vi "PC_AINoiseMeas.vi"() -> ()   [LabVIEW 2020]
uses:
  TypeDefs/UIStateDefEnum.ctl
  <vilib>/measure/maspectr.llb/Power Spectrum and PSD Export Mode.ctl
  <vilib>/Analysis/baseanly.llb/Mean (DBL).vi
  <vilib>/Analysis/5stat.llb/RMS (DBL).vi
  <vilib>/NI/STM/TCP/Read Meta Data (TCP Ref).vi
  <vilib>/NI/STM/TCP/Get Connection Reference (TCP).vi
  <vilib>/measure/maspectr.llb/FFT Power Spectrum and PSD for 1 Chan.vi
  <vilib>/Analysis/1siggen.llb/Ramp Pattern by Delta.vi
  <vilib>/Utility/file.llb/Write Delimited Spreadsheet (DBL).vi
  <vilib>/NI/STM/TCP/Read Meta Data (TCP Clst).vi
  <vilib>/NI/STM/TCP/Read Message (TCP).vi
  <vilib>/NI/STM/NI STM.lvlib
  <vilib>/Analysis/NI_AALBase.lvlib
  <vilib>/measure/NI_MAPro.lvlib
  <vilib>/Analysis/NI_AALPro.lvlib
  Components_global/Spectra/Spectra.lvlib
panel:
  in  "STM LoopTime Set [ms]":u32=100
  in  "Save Data":bool
  out "Analysis Loop \ntime [s]":dbl format="%#.4g"
  out "Analysis \ntime-span [s]":dbl format="%.2f"
  out "# of elements \nremoved":i32
  in  "Pause Charts":bool
  in  "Clear charts":bool
  out "RT target \nloop \ntime [s]":dbl=0.0002
  out "Data length \n[count]":i32
  out "Mean [V]":dbl format="%#.6f"
  out "RMS / \nStd. Dev. [mV]":dbl format="%#.6f"
  out "Spectra plots":cluster{"f0":dbl, "df":dbl, "magnitude":dbl[]}[](graph)
  out "Histogram Graph":T1(graph)
  out "STM Loop \ntime [s]":dbl format="%#.4g"
  in  "System Stop Button":bool
  out "Data":dbl[][](graph)
  # "Hidden Controls and Indicators"
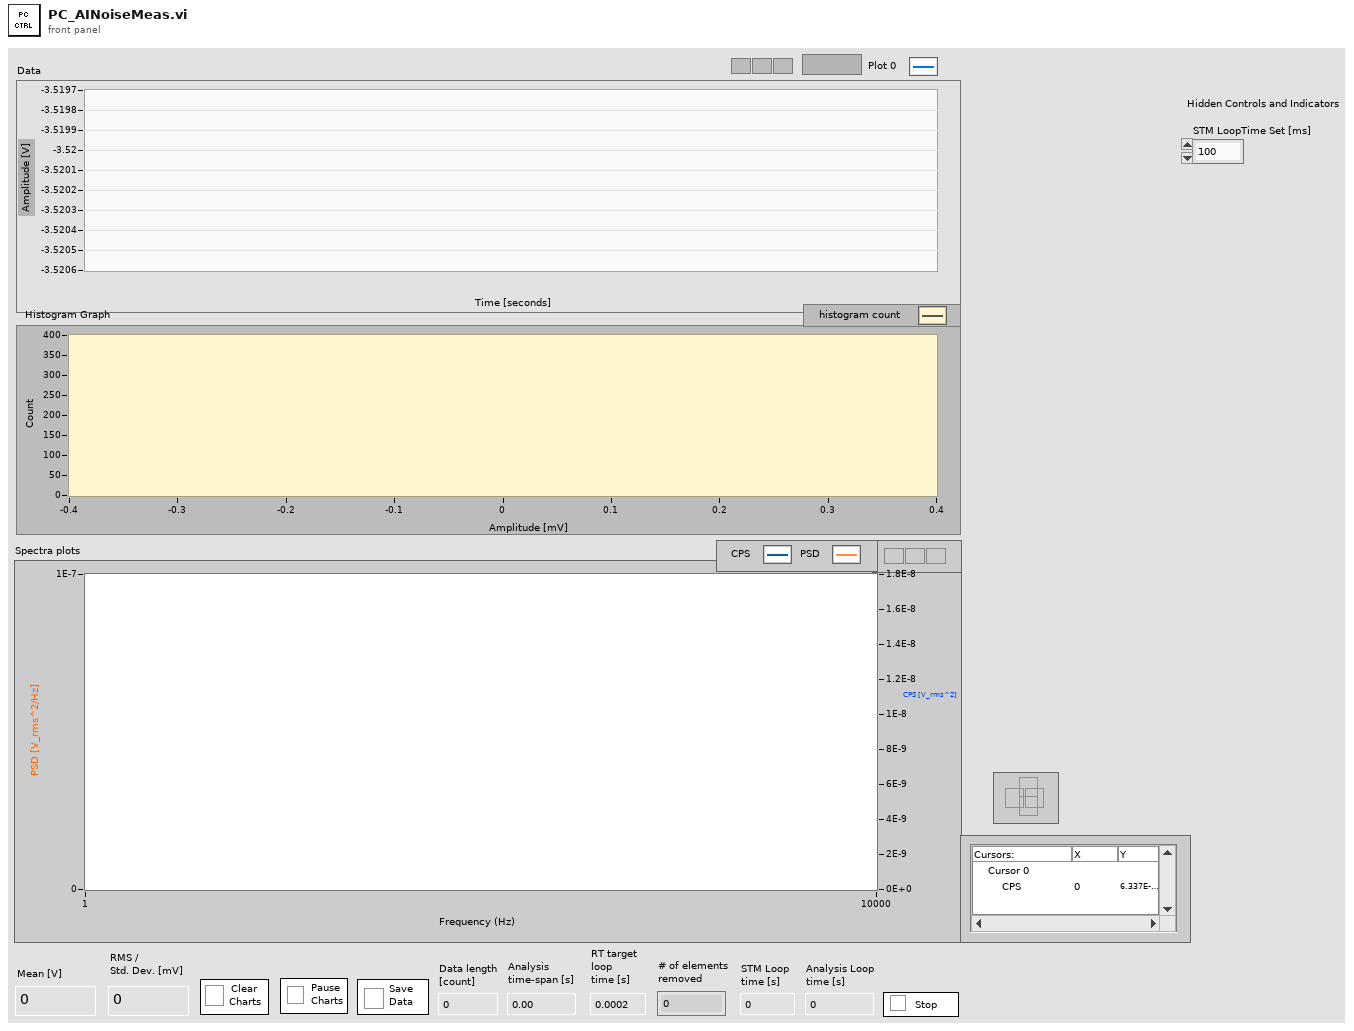
[diagram p1: front panel]
types:
  T1 = cluster{"X Values":dbl[], "Histogram: h(x)":i32[]}
  T2 = typedef "UIStateDefEnum.ctl" = enum16{"Wait", "Initialize", "Clear", "SaveData", "Stop"}
  T3 = typedef "NI STM.lvlib/TCP Connection Info.ctl" = cluster{"connection ID":refnum<k5>, "meta data":T4[]}
  T4 = typedef "NI STM.lvlib/MetaDataElement.ctl" = string
  T5 = typedef "NI_MAPro.lvlib/Power Spectrum and PSD Export Mode.ctl" = u16
  T6 = typedef "imagedata.ctl" = cluster{"image type":i32, "image depth":i32, "image":u8[], "mask":u8[], "colors":u32[], "Rectangle":cluster{"left":i16, "top":i16, "right":i16, "bottom":i16}}
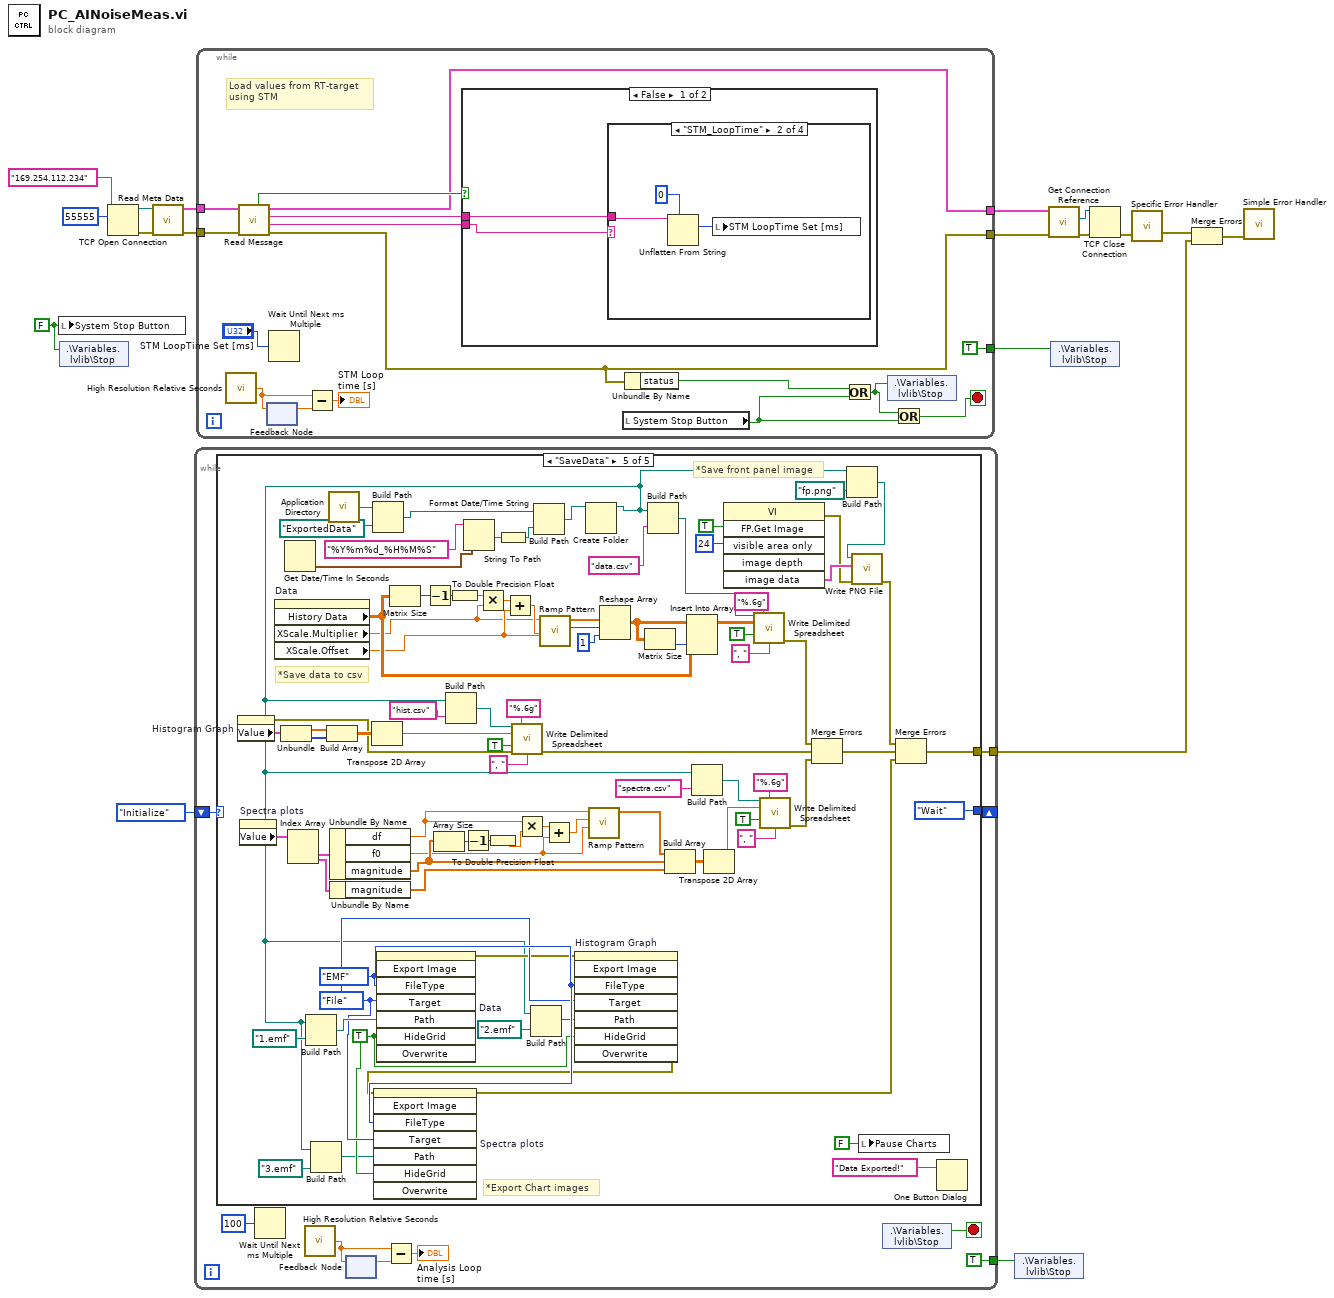
[diagram p0: block diagram]
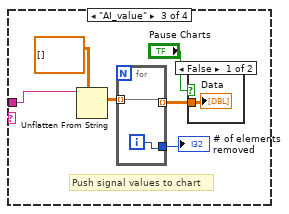
[diagram p3: hidden frame]
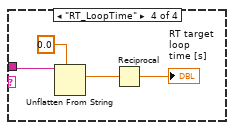
[diagram p5: hidden frame]
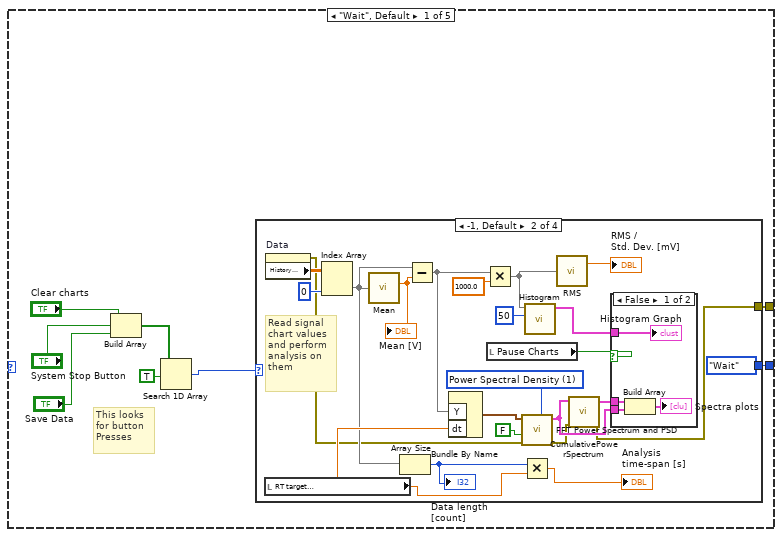
[diagram p7: hidden frame]
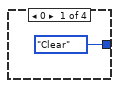
[diagram p8: hidden frame]
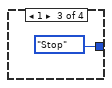
[diagram p10: hidden frame]
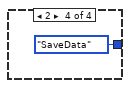
[diagram p11: hidden frame]
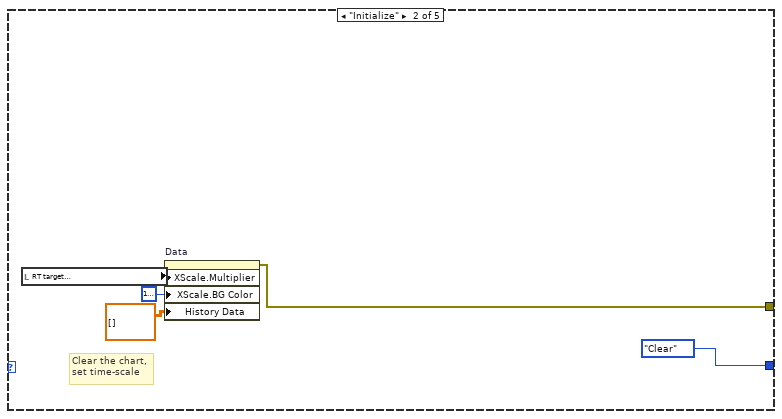
[diagram p12: hidden frame]
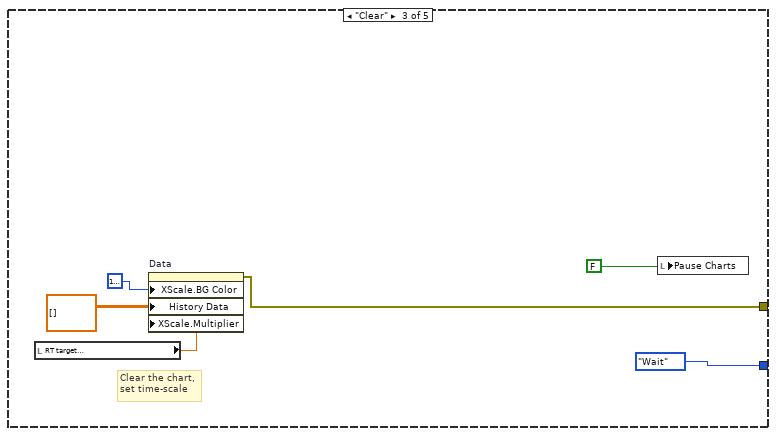
[diagram p13: hidden frame]
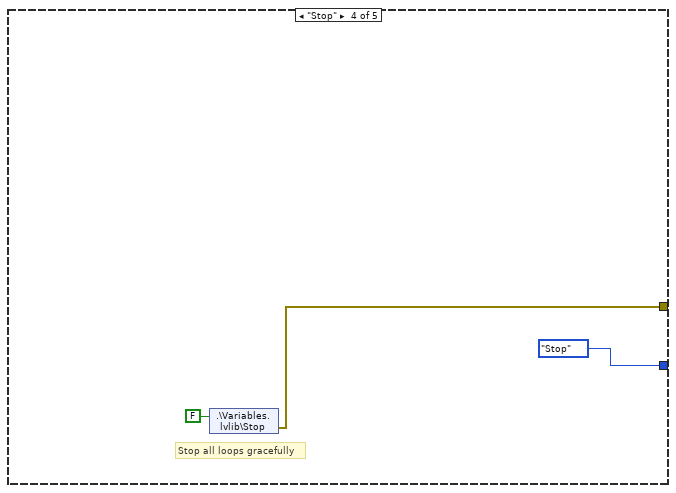
[diagram p14: hidden frame]
diagram:
  w7 = FALSE ("System Stop Button")
  n1 = local write "System Stop Button"(w7) -> ()
  n2 = shared-variable ".\\Variables.lvlib\\Stop"(w7) -> ()  [unwired: 1 in, 1 out]
  n3 = TCP Open Connection(address="169.254.112.234", remote port or service name=u16 55555) -> (connection ID=w16:refnum<k5>, error out=w15:errorcluster)  [unwired: 3 in]
  n4 = call-poly <vilib>:"Read Meta Data.vi"("error in"=w15, "connection ID"=w16) -> ("error out"=w13:errorcluster, "connection info out"=w14:T3)  [unwired: 7 in, 1 out]
  n5 = while {
    shift-right: [w25] -> _
    shift-left: UIStateDefEnum."Initialize" ("UIStateDefEnum") -> [w26]
    tunnel: [w20] -> w2
    tunnel: [TRUE ("Stop")] -> w1
    stop <- w24 stop-if-true
    n6 = case shown="\"SaveData\"" w26 {
      tunnel: [w30 UIStateDefEnum."Clear" ("UIStateDefEnum") UIStateDefEnum."Wait" ("UIStateDefEnum") UIStateDefEnum."Stop" ("UIStateDefEnum") UIStateDefEnum."Wait" ("UIStateDefEnum")] -> w25
      tunnel: [w28 w66 w71 w77 w120] -> w20
      frame "Wait", Default {
        # "This looks \nfor button \nPresses"
        n7 = Build Array "Build Array"("Clear charts", "System Stop Button", "Save Data") -> (w35:bool[])
        n8 = Search 1D Array(1D array=w35, element=TRUE) -> (index of element=w31:i32)  [unwired: 1 in]
        n9 = case shown="-1, Default" w31 {
          tunnel: [UIStateDefEnum."Clear" ("UIStateDefEnum") UIStateDefEnum."Wait" ("UIStateDefEnum") UIStateDefEnum."Stop" ("UIStateDefEnum") UIStateDefEnum."SaveData" ("UIStateDefEnum")] -> w30
          tunnel: [_ w37 _ _] -> w28
          frame 0 {
          }
          frame -1, Default {
            w55 = T5 1 items=["Power Spectrum", "Power Spectral Density"] ("export mode")
            # "Read signal\nchart values\nand perform\nanalysis on \nthem"
            n10 = local read "RT target \nloop \ntime [s]"() -> (w48:dbl)
            n11 = property on="Data" class="WFChart (strict)"() -> (error out=w38:errorcluster, "History Data"=w53:dbl[][])  [unwired: 2 in, 1 out]
            n12 = Index Array(array=w53, index (col)=0 ("disabled index (col)")) -> (element=w43:dbl[])  [unwired: 1 in]
            n13 = call-poly <vilib>:"Mean.vi"("X"=w43) -> ("mean"=w54:dbl)  [unwired: 1 out]
            "Mean [V]" <- w54
            n14 = Array Size(array=w43) -> (size(s)=w49:i32)
            "Data length \n[count]" <- w49
            n15 = Subtract(x=w43, y=w54) -> (x-y=w42:dbl[])
            n16 = Bundle By Name("Y"=w42, "dt"=w48) -> (w57:waveform(dbl))  [unwired: 1 in]
            n17 = Multiply(x=w42, y=1000.0) -> (x*y=w44:dbl[])
            n18 = local read "Pause Charts"() -> (w47:bool)
            n19 = call-poly <vilib>:"FFT Power Spectrum and PSD.vi"("export mode"=w55, "error in (no error)"=w38, "dB On (F)"=FALSE, "time signal"=w57) -> ("error out"=w39:errorcluster, "Power Spectrum / PSD"=w40:cluster{"f0":dbl, "df":dbl, "magnitude":dbl[]})  [unwired: 4 in, 2 out]
            n20 = Multiply(x=w49, y=w48) -> (x*y=→"Analysis \ntime-span [s]":dbl)
            n21 = call <vilib>:"Histogram.vi"("intervals"=50, "X"=w44) -> ("Histogram Graph"=w58:T1)  [unwired: 6 in, 3 out]
            n22 = call-poly <vilib>:"RMS.vi"("X"=w44) -> ("rms value"=→"RMS / \nStd. Dev. [mV]":dbl)  [unwired: 1 out]
            n23 = call "CumulativePowerSpectrum.vi"("error in (no error)"=w39, "PSD"=w40) -> ("error out"=w37:errorcluster, "CPS"=w41:cluster{"f0":dbl, "df":dbl, "magnitude":dbl[]})  [unwired: 8 in]
            n24 = case shown="False" w47 {
              tunnel: w58 -> [w63 _]
              tunnel: w41 -> [w62 _]
              tunnel: w40 -> [w60 _]
              frame False {
                n25 = Build Array(w62, w60) -> (→"Spectra plots":cluster{"f0":dbl, "df":dbl, "magnitude":dbl[]}[])
                "Histogram Graph" <- w63
              }
              frame True {
              }
            }
          }
          frame 1 {
          }
          frame 2 {
          }
        }
      }
      frame "Initialize" {
        # "Clear the chart,\nset time-scale"
        n26 = local read "RT target \nloop \ntime [s]"() -> (w69:dbl)
        n27 = property on="Data" class="WFChart (strict)"("XScale.Multiplier"=w69, "XScale.BG Color"=u32 16777216 ("X Scale.Marker Colors:BG Color"), "History Data"=dbl[][] []) -> (error out=w66:errorcluster)  [unwired: 2 in, 1 out]
      }
      frame "Clear" {
        # "Clear the chart,\nset time-scale"
        n28 = local read "RT target \nloop \ntime [s]"() -> (w72:dbl)
        n29 = property on="Data" class="WFChart (strict)"("XScale.BG Color"=u32 16777216 ("X Scale.Marker Colors:BG Color"), "History Data"=dbl[][] [], "XScale.Multiplier"=w72) -> (error out=w71:errorcluster)  [unwired: 2 in, 1 out]
        n30 = local write "Pause Charts"(FALSE ("Pause Charts")) -> ()
      }
      frame "Stop" {
        # "Stop all loops gracefully"
        n31 = shared-variable ".\\Variables.lvlib\\Stop"(FALSE ("Stop")) -> (error out=w77:errorcluster)  [unwired: 1 in]
      }
      frame "SaveData" {
        w133 = TRUE ("Hide Grid")
        w136 = enum32{"File", "Clipboard"}."File" ("Target")
        w137 = enum32{"BMP", "EPS", "EMF", "PICT"}."EMF" ("File Type")
        # "*Export Chart images"
        # "*Save front panel image"
        # "*Save data to csv"
        n32 = property on="Histogram Graph" class="XYGraph (strict)"() -> (error out=w91:errorcluster, "Value"=w117:T1)  [unwired: 2 in, 1 out]
        n33 = property on="Spectra plots" class="WFGraph (strict)"() -> ("Value"=w113:cluster{"f0":dbl, "df":dbl, "magnitude":dbl[]}[])  [unwired: 2 in, 2 out]
        n34 = property on="Data" class="WFChart (strict)"() -> ("History Data"=w161:dbl[][], "XScale.Multiplier"=w151:dbl, "XScale.Offset"=w156:dbl)  [unwired: 2 in, 2 out]
        n35 = Unbundle(w117) -> ("X Values"=w116:dbl[], "Histogram: h(x)"=w115:i32[])
        n36 = Get Date/Time In Seconds() -> (seconds since 1Jan1904=w148:timestamp)
        n37 = Index Array(array=w113) -> (element #1=w112:cluster{"f0":dbl, "df":dbl, "magnitude":dbl[]}, element #2=w111:cluster{"f0":dbl, "df":dbl, "magnitude":dbl[]})  [unwired: 2 in]
        n38 = Build Array(w116, w115) -> (w114:dbl[][])
        n39 = call <vilib>:"Application Directory.vi"() -> ("Application Directory"=w150:path)
        n40 = Unbundle By Name(w112) -> ("df"=w105:dbl, "f0"=w103:dbl, "magnitude"=w108:dbl[])
        n41 = Unbundle By Name(w111) -> ("magnitude"=w110:dbl[])
        n42 = Transpose 2D Array(2D array=w114) -> (transposed array=w92:dbl[][])
        n43 = Build Path(base path=w150, name or relative path=path "ExportedData") -> (appended path=w145:path)
        n44 = Matrix Size(0:w161) -> (1:w160:i32)  [unwired: 1 out]
        n45 = Decrement(x=w160) -> (x-1=w159:i32)
        n46 = Array Size(array=w108) -> (size(s)=w100:i32)
        n47 = To Double Precision Float(number=w159) -> (double precision float=w158:dbl)
        n48 = Decrement(x=w100) -> (x-1=w107:i32)
        n49 = Format Date/Time String(time format string (%c)="%Y%m%d_%H%M%S", seconds (now)=w148) -> (date/time string=w143:string)  [unwired: 1 in]
        n50 = Multiply(x=w158, y=w151) -> (x*y=w157:dbl)
        n51 = To Double Precision Float(number=w107) -> (double precision float=w106:dbl)
        n52 = String To Path(string=w143) -> (path=w144:path)
        n53 = Add(x=w157, y=w156) -> (x+y=w155:dbl)
        n54 = Multiply(x=w105, y=w106) -> (x*y=w104:dbl)
        n55 = Build Path(base path=w145, name or relative path=w144) -> (appended path=w138:path)
        n56 = call-poly <vilib>:"Ramp Pattern.vi"("start"=w156, "end"=w155, "delta"=w151) -> ("samples"=w154:i32, "Ramp Pattern"=w153:dbl[])  [unwired: 6 in, 1 out]
        n57 = Add(x=w104, y=w103) -> (x+y=w102:dbl)
        n58 = Create Folder(path (use dialog)=w138) -> (created path=w82:path)  [unwired: 2 in, 2 out]
        n59 = Build Path(base path=w82, name or relative path=path "1.emf") -> (appended path=w141:path)
        n60 = Build Path(base path=w82, name or relative path=path "3.emf") -> (appended path=w132:path)
        n61 = invoke on="Data" class="WFChart (strict)" method="Export Image"("FileType"=w137, "Target"=w136, "Path"=w141, "HideGrid"=w133) -> (error out=w130:errorcluster)  [unwired: 4 in, 7 out]
        n62 = Build Path(base path=w82, name or relative path="hist.csv" ("string")) -> (appended path=w93:path)
        n63 = call-poly <vilib>:"Write Delimited Spreadsheet.vi"("file path (dialog if empty)"=w93, "format (%.3f)"="%.6g", "2D data"=w92, "append to file? (new file:F)"=TRUE, "error in (no error)"=w91, "delimiter (\\t)"=", " ("delimiter (\\t)")) -> ("error out"=w89:errorcluster)  [unwired: 8 in, 1 out]
        n64 = Build Path(base path=w82, name or relative path=path "2.emf") -> (appended path=w135:path)
        n65 = invoke on="Histogram Graph" class="XYGraph (strict)" method="Export Image"(error in=w130, "FileType"=w137, "Target"=w136, "Path"=w135, "HideGrid"=w133) -> (error out=w129:errorcluster)  [unwired: 3 in, 7 out]
        n66 = invoke on="Spectra plots" class="WFGraph (strict)" method="Export Image"(error in=w129, "FileType"=w137, "Target"=w136, "Path"=w132, "HideGrid"=w133) -> (error out=w109:errorcluster)  [unwired: 3 in, 7 out]
        n67 = call-poly <vilib>:"Ramp Pattern.vi"("start"=w103, "end"=w102, "delta"=w105) -> ("Ramp Pattern"=w101:dbl[])  [unwired: 6 in, 2 out]
        n68 = Reshape Array(w153, w154, 1 ("dimension size")) -> (w152:dbl[][])
        n69 = Matrix Size(0:w152) -> (2:w163:i32)  [unwired: 1 out]
        n70 = Build Path(base path=w82, name or relative path="data.csv" ("string")) -> (appended path=w146:path)
        n71 = Build Array(w101, w108, w110) -> (w99:dbl[][])
        n72 = Insert Into Array(array=w152, index (col)=w163, new element=w161) -> (w98:dbl[][])  [unwired: 1 in]
        n73 = Build Path(base path=w82, name or relative path="spectra.csv" ("string")) -> (appended path=w87:path)
        n74 = Transpose 2D Array(2D array=w99) -> (transposed array=w81:dbl[][])
        n75 = invoke class="VI" method="FP.Get Image"("visible area only"=TRUE ("Visible Area Only"), "image depth"=24 ("Image Depth")) -> (error out=w124:errorcluster, "image data"=w126:T6)  [unwired: 4 in, 4 out]
        n76 = call-poly <vilib>:"Write Delimited Spreadsheet.vi"("file path (dialog if empty)"=w146, "format (%.3f)"="%.6g", "2D data"=w98, "append to file? (new file:F)"=TRUE, "delimiter (\\t)"=", " ("delimiter (\\t)")) -> ("error out"=w90:errorcluster)  [unwired: 9 in, 1 out]
        n77 = call-poly <vilib>:"Write Delimited Spreadsheet.vi"("file path (dialog if empty)"=w87, "format (%.3f)"="%.6g", "2D data"=w81, "append to file? (new file:F)"=TRUE, "delimiter (\\t)"=", " ("delimiter (\\t)")) -> ("error out"=w80:errorcluster)  [unwired: 9 in, 1 out]
        n78 = Merge Errors(w90, w89, w80) -> (w88:errorcluster)
        n79 = Build Path(base path=w82, name or relative path=path "fp.png") -> (appended path=w125:path)
        n80 = call <vilib>:"Write PNG File.vi"("error in (no error)"=w124, "image data"=w126, "path to PNG file"=w125) -> ("error out"=w122:errorcluster)  [unwired: 7 in, 1 out]
        n81 = local write "Pause Charts"(FALSE ("Pause Charts")) -> ()
        n82 = Merge Errors(w122, w88, w109) -> (w120:errorcluster)
        n83 = One Button Dialog(message="Data Exported!" ("Status....")) -> ()  [unwired: 1 in, 1 out]
      }
    }
    n84 = Wait Until Next ms Multiple(millisecond multiple=u32 100) -> ()  [unwired: 1 out]
    n85 = call <vilib>:"High Resolution Relative Seconds.vi"() -> ("relative seconds"=w22:dbl)
    n86 = feedback #1() -> (w23:dbl)  [unwired: 1 in]
    n87 = feedback-in #1(w22) -> ()
    n88 = Subtract(x=w22, y=w23) -> (x-y=→"Analysis Loop \ntime [s]":dbl)
    n89 = shared-variable ".\\Variables.lvlib\\Stop"() -> (w24:bool)  [unwired: 1 in, 1 out]
  }
  n90 = while {
    tunnel: w14 -> [w181]
    tunnel: w13 -> [w180]
    tunnel: [w178] -> w9
    tunnel: [w177] -> w8
    tunnel: [TRUE ("Stop")] -> w5
    stop <- w171 stop-if-true
    # "Load values from RT-target\nusing STM"
    n91 = call <vilib>:"High Resolution Relative Seconds.vi"() -> ("relative seconds"=w173:dbl)
    n92 = call-poly <vilib>:"Read Message.vi"("error in"=w180, "connection info in"=w181) -> ("error out"=w177:errorcluster, "name"=w176:T4, "data string"=w175:string, "connection info out"=w178:T3, "timed out?"=w179:bool)  [unwired: 4 in, 1 out]
    n93 = feedback-in #2(w173) -> ()
    n94 = feedback #2() -> (w174:dbl)  [unwired: 1 in]
    n95 = Wait Until Next ms Multiple(millisecond multiple="STM LoopTime Set [ms]") -> ()  [unwired: 1 out]
    n96 = Subtract(x=w173, y=w174) -> (x-y=→"STM Loop \ntime [s]":dbl)
    n97 = case shown="False" w179 {
      tunnel: w176 -> [w183 _]
      tunnel: w175 -> [w182 _]
      frame False {
        n98 = case shown="\"STM_LoopTime\"" w183 {
          tunnel: w182 -> [_ w185 w191 w196]
          frame Default {
          }
          frame "STM_LoopTime" {
            n99 = Unflatten From String(type=u32 0, binary string=w185) -> (value=w184:u32)  [unwired: 3 in, 2 out]
            n100 = local write "STM LoopTime Set [ms]"(w184) -> ()
          }
          frame "AI_value" {
            # "Push signal values to chart"
            n101 = Unflatten From String(type=dbl[][] [], binary string=w191) -> (value=w190:dbl[][])  [unwired: 3 in, 2 out]
            n102 = for {
              tunnel: w190 -> [w195] mode=indexing
              tunnel: [w195] -> w189 mode=indexing
              tunnel: [w194] -> w188
              i -> [w194]
            }
            "# of elements \nremoved" <- w188
            n103 = case shown="False" "Pause Charts" {
              tunnel: w189 -> [w193 _]
              frame False {
                "Data" <- w193
              }
              frame True {
              }
            }
          }
          frame "RT_LoopTime" {
            n104 = Unflatten From String(type=0.0, binary string=w196) -> (value=w198:dbl)  [unwired: 3 in, 2 out]
            n105 = Reciprocal(x=w198) -> (1/x=→"RT target \nloop \ntime [s]":dbl)
          }
        }
      }
      frame True {
      }
    }
    n106 = local read "System Stop Button"() -> (w170:bool)
    n107 = Unbundle By Name(w177) -> ("status"=w169:bool)
    n108 = Or(x=w169, y=w170) -> (x .or. y?=w168:bool)
    n109 = shared-variable ".\\Variables.lvlib\\Stop"(w168) -> ()  [unwired: 1 in, 1 out]
    n110 = Or(x=w168, y=w170) -> (x .or. y?=w171:bool)
  }
  n111 = shared-variable ".\\Variables.lvlib\\Stop"(w1) -> ()  [unwired: 1 in, 1 out]
  n112 = call-poly <vilib>:"Get Connection Reference.vi"("error in"=w8, "connection info in"=w9) -> ("error out"=w12:errorcluster, "connection ID out"=w11:refnum<k5>)  [unwired: 7 in, 1 out]
  n113 = shared-variable ".\\Variables.lvlib\\Stop"(w5) -> ()  [unwired: 1 in, 1 out]
  n114 = TCP Close Connection(connection ID=w11, error in (no error)=w12) -> (error out=w10:errorcluster)  [unwired: 1 in, 1 out]
  n115 = call "Specific Error Handler"("Error to Check"=w10) -> ("error out"=w4:errorcluster)  [unwired: 11 in, 3 out]
  n116 = Merge Errors(w4, w2) -> (w3:errorcluster)
  n117 = call <vilib>:"Simple Error Handler.vi"("error in (no error)"=w3) -> ()  [unwired: 4 in, 5 out]
